vi "calculate torque start.vi"() -> ()   [LabVIEW 2019]
doc: "This vi will take two forces and two moments and do the cross product to get torque vector.\n\nJuan Gamez\nP3600"
uses:
  typedefs/moment arm vector.ctl
  typedefs/force vector.ctl
  P2 sol pw/typedefs/torque vector.ctl
panel:
  out "Resultant Torque":T1
  in  "Force B":T2={"Fx"=0.0, "Fy"=0.0, "Fz"=10.0}
  in  "Force A":T2={"Fx"=0.0, "Fy"=10.0, "Fz"=0.0}
  in  "Moment Arm B":T3={"Rx"=0.0, "Ry"=10.0, "Rz"=0.0}
  in  "Moment Arm A":T3={"Rx"=10.0, "Ry"=0.0, "Rz"=0.0}
  # "Calculating Torques\nJuan Gamez\nP3600"
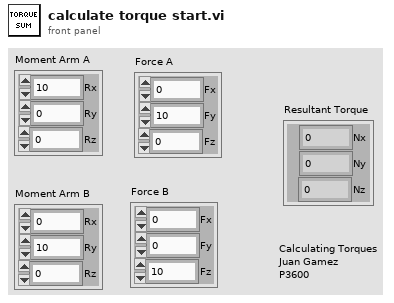
[diagram p1: front panel]
types:
  T1 = typedef "torque vector.ctl" = cluster{"Nx":dbl, "Ny":dbl, "Nz":dbl}
  T2 = typedef "force vector.ctl" = cluster{"Fx":dbl, "Fy":dbl, "Fz":dbl}
  T3 = typedef "moment arm vector.ctl" = cluster{"Rx":dbl, "Ry":dbl, "Rz":dbl}
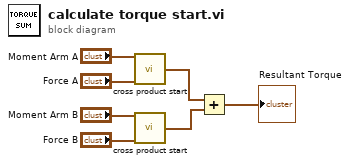
[diagram p0: block diagram]
diagram:
  n1 = call "cross product start.vi"("Moment Arm"="Moment Arm A", "Force"="Force A") -> ("Torque  Vector"=w2:T1)  [unwired: 13 in]
  n2 = call "cross product start.vi"("Moment Arm"="Moment Arm B", "Force"="Force B") -> ("Torque  Vector"=w1:T1)  [unwired: 13 in]
  n3 = Add(x=w2, y=w1) -> (x+y=→"Resultant Torque":T1)
